vi "USRP DUP.vi"() -> ()   [LabVIEW 2014]
uses:
  <instrlib>/niUSRP/niUSRP Write Tx Data (CDB WDT).vi
  <vilib>/measure/NI_MABase.lvlib
panel:
  in  "channel list":string
  in  "signal type":T1(ring)
  in  "square wave duty cycle (%)":dbl=50.0 format="%0.2f"
  out "Waveform Graph":waveform(dbl)(graph)
  in  "Boolean":bool
  in  "frequency":dbl=10.0 format="%0.2p"
  in  "active antenna":string
  in  "carrier frequency":dbl=100000.0 format="%#_6p"
  in  "IQ rate":dbl=100000.0 format="%#_6p"
  in  "device names":refnum<k15>
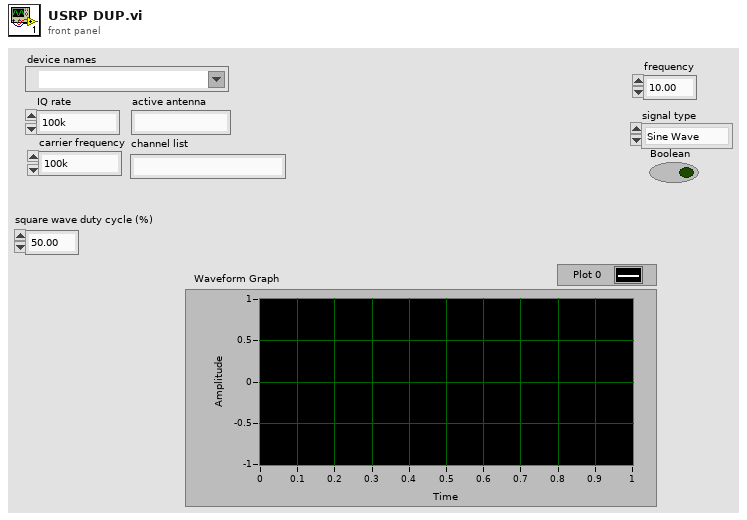
[diagram p1: front panel]
types:
  T1 = enum16{"Sine Wave", "Triangle Wave", "Square Wave", "Sawtooth Wave"}
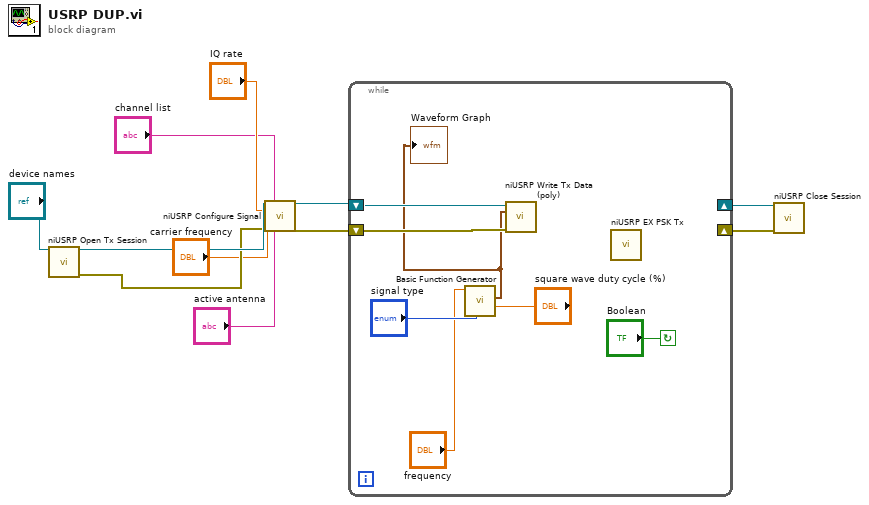
[diagram p0: block diagram]
diagram:
  n1 = call <instrlib>:"niUSRP Open Tx Session.vi"("device names"="device names") -> ("session handle out"=w10:refnum<k15>, "error out"=w9:errorcluster)  [unwired: 13 in]
  n2 = call <instrlib>:"niUSRP Configure Signal.vi"("session handle"=w10, "channel list"="channel list", "IQ rate"="IQ rate", "carrier frequency"="carrier frequency", "error in (no error)"=w9, "active antenna"="active antenna") -> ("session handle out"=w8:refnum<k15>, "error out"=w7:errorcluster)  [unwired: 5 in, 3 out]
  n3 = while {
    shift-right: [_] -> w6
    shift-left: w8 -> [w19]
    shift-right: [_] -> w5
    shift-left: w7 -> [w18]
    stop <- "Boolean" continue-if-true
    n4 = call <vilib>:"Basic Function Generator.vi"("square wave duty cycle (%)"="square wave duty cycle (%)", "signal type"="signal type", "frequency"="frequency") -> ("signal out"=w13:waveform(dbl))  [unwired: 6 in, 2 out]
    "Waveform Graph" <- w13
    n5 = call-poly <instrlib>:"niUSRP Write Tx Data (poly).vi"("session handle"=w19, "data"=w13, "error in (no error)"=w18) -> ("error out"=w12:errorcluster)  [unwired: 11 in, 1 out]
    n6 = call "niUSRP EX PSK Tx.vi"() -> ()  [unwired: 1 in]
  }
  n7 = call <instrlib>:"niUSRP Close Session.vi"("session handle"=w6, "error in (no error)"=w5) -> ()  [unwired: 13 in, 1 out]
